vi "getCorners.vi"(8 "error in (no error)":errorcluster, 11 "StationKeeping in":refnum<class "StationKeeping.lvclass">) -> (0 "error out":errorcluster, 2 "output array":T1[](array[typedef]) {"North" format="%#_10f"; "East" format="%#_8f"}, 3 "StationKeeping out":refnum<class "StationKeeping.lvclass">)   [LabVIEW 2013, in "StationKeeping.lvclass"]
doc: "Returns the four corners of the station keeping box in no particular order\n\nAssumes the station keeping box is square\nBox can be at any arbitrary angle"
uses:
  StationKeeping.lvclass
  Data/TypeDefs/UTM Location.ctl
  <vilib>/imath/engines/lvmath2/RunTimeEngine/ErrorHandling/NIMS_Finalize Error.vi
  <vilib>/imath/engines/lvmath2/RunTimeEngine/Managers/WorkSpace/UID Generator.vi
  <vilib>/imath/engines/lvmath2/RunTimeEngine/Managers/SymbolTable/Clear UID.vi
  <vilib>/imath/engines/lvmath2/RunTimeEngine/NodeEndStatement/NIMS_NodeEndStatement_Output.vi
  <instcachedir>/0/NIMS_NodeEndStatement_Output_53EC0D466D134D7ABD903AC30B43404B.lvgen/NIMS_NodeEndStatement_Output_53EC0D466D134D7ABD903AC30B43404B_001.vi
  <vilib>/imath/engines/lvmath2/RunTimeEngine/RunTimeType/NIMS_RunTimeType_From StrictType (excl LVString).vi
  <instcachedir>/0/NIMS_RunTimeType_From StrictType (excl LVString)_4DEE718D6EB74582AA20236969C084FC.lvgen/NIMS_RunTimeType_From StrictType (excl LVString)_4DEE718D6EB74582AA20236969C084FC_000.vi
  <vilib>/imath/engines/lvmath2/RunTimeEngine/LocalVariableDefStatement/MC_LocalVariableDefStatement_Display.vi
  <vilib>/imath/engines/lvmath2/RunTimeEngine/Managers/SymbolTable/NIMS_WorkSpace.lvlib
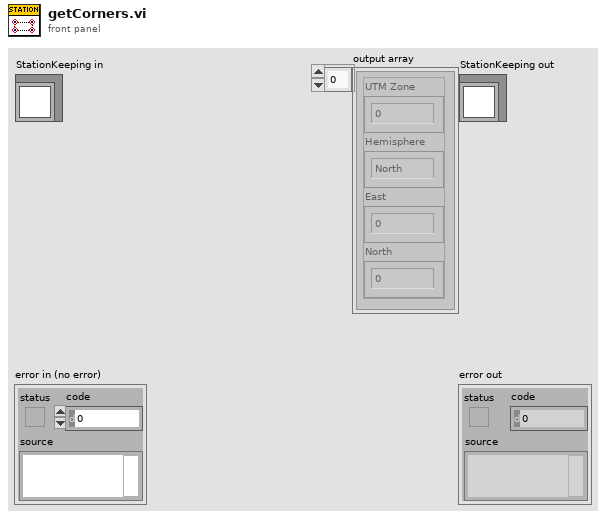
[diagram p1: front panel]
types:
  T1 = typedef "UTM Location.ctl" = cluster{"UTM Zone":dbl, "Hemisphere":enum16{"North", "South"}, "East":dbl, "North":dbl}
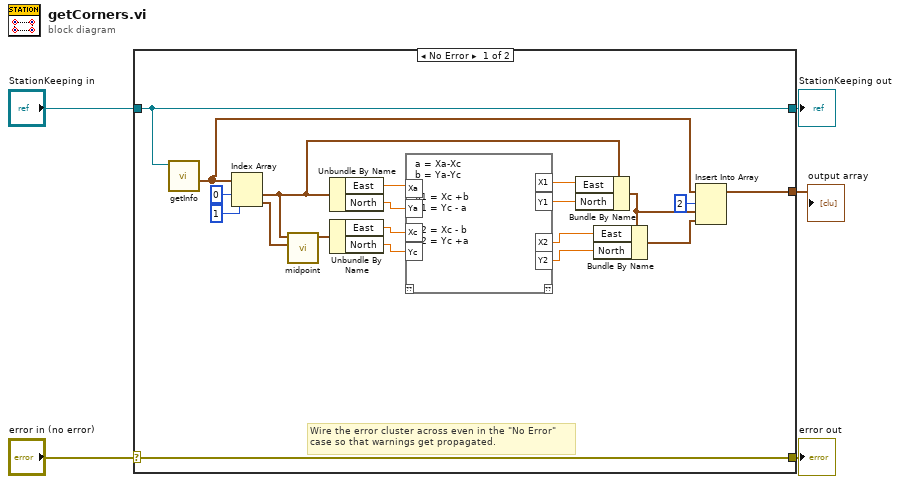
[diagram p0: block diagram]
diagram:
  n1 = case shown="No Error" "error in (no error)" {
    selector: "error in (no error)" -> [w25 w150]
    tunnel: [w25 w150] -> w4
    tunnel: [w24 w149] -> w2
    tunnel: "StationKeeping in" -> [w24 w149]
    tunnel: [w14 _] -> w1
    frame No Error {
      # "Wire the error cluster across even in the \"No Error\"\ncase so that warnings get propagated."
      n2 = call-dynamic "getInfo.vi"("GenericMission in"=w24) -> ("Points of Interest"=w18:T1[])  [unwired: 3 in, 7 out]
      n3 = Index Array(array=w18, index #1=0 ("index"), index #2=1 ("index")) -> (element #1=w19:T1, element #2=w21:T1)
      n4 = call "midpoint.vi"("UTM Location 2"=w21, "UTM Location"=w19) -> ("UTM Location 3"=w20:T1)  [unwired: 8 in, 1 out]
      n5 = Unbundle By Name(w19) -> ("East"=w13:dbl, "North"=w12:dbl)
      n6 = Unbundle By Name(w20) -> ("East"=w11:dbl, "North"=w10:dbl)
      n7 = mathscript code="a = Xa-Xc\nb = Ya-Yc\n\nX1 = Xc +b\nY1 = Yc - a\n\nX2 = Xc - b\nY2 = Yc +a"("Xa"=w13, "Ya"=w12, "Xc"=w11, "Yc"=w10) -> ("X1"=w9:dbl, "X2"=w7:dbl, "Y1"=w8:dbl, "Y2"=w6:dbl)  [unwired: 1 in, 1 out]
      n8 = Bundle By Name(cluster=w19, "East"=w9, "North"=w8) -> (w17:T1)
      n9 = Bundle By Name(cluster=w17, "East"=w7, "North"=w6) -> (w16:T1)
      n10 = Insert Into Array(array=w18, index=2, new element #1=w17, new element #2=w16) -> (w14:T1[])
    }
    frame Error {
    }
  }
  "error out" <- w4
  "StationKeeping out" <- w2
  "output array" <- w1
